vi "duplicate channel.vi"(8 "number of available channels":u16, 11 "Sensor List":u32) -> (2 "Sensor Array out":T1, 3 "IndexVals":u32)   [LabVIEW 2015]
uses:
  DAQ configuration/Sensor array.ctl
  DAQ configuration/channel identifier.ctl
  DAQ configuration/Sensor buffer command.ctl
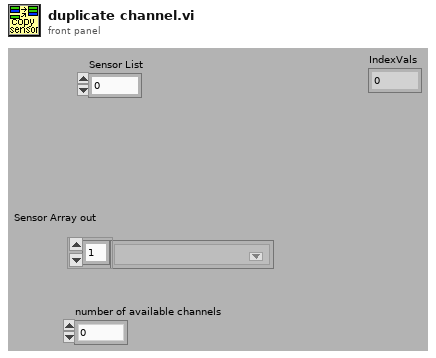
[diagram p1: front panel]
types:
  T1 = typedef "Sensor array.ctl" = T2[]
  T2 = typedef "channel identifier.ctl" = u16
  T3 = typedef "Sensor buffer command.ctl" = enum16{"read average", "read recent", "read all", "write", "set buffer size", "Read channel config", "Write channel config", "clear"}
  T4 = typedef "Channel config.ctl" = cluster{"Channel Indices":T2[], "AI Max voltage":dbl[], "Calibration matrix":T5}
  T5 = typedef "calib array.ctl" = T6[]
  T6 = typedef "conversion.ctl" = cluster{"conversion matrix":sgl[][], "units":string, "name":string, "scale type":T7, "offset (volts)":dbl, "second channel":i8, "correspondence table":T8, "offset (physical units)":dbl, "pH scale":T9, "D.O.":T10, "Photometer data":T11}
  T7 = typedef "scale type.ctl" = enum16{"Volts", "Polynomial", "Correspondence Table", "pH", "Dissolved Oxygen", "Quadratic", "Photometer"}
  T8 = typedef "correspondence table.ctl" = cluster{"physical units":dbl, "volts":dbl}[]
  T9 = typedef "pH scale.ctl" = cluster{"Buffers":cluster{"Buffer":dbl, "Calibrated":bool, "V/T":dbl}[], "Temperature":dbl}
  T10 = typedef "DO scale.ctl" = cluster{"Temperature":dbl, "K":dbl, "barometric pressure":dbl}
  T11 = typedef "Photometer calibration data.ctl" = cluster{"Dark Voltage":dbl, "Blank Voltage":dbl, "Standards":cluster{"Concentration":dbl, "Voltage":dbl}[]}
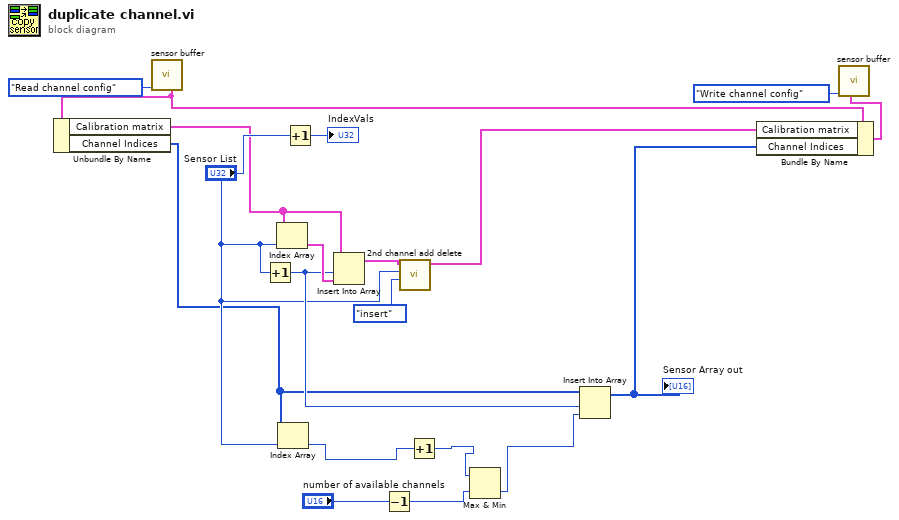
[diagram p0: block diagram]
diagram:
  n1 = call "sensor buffer.vi"("command"=Sensor_buffer_command."Read channel config") -> ("Channel Config out"=w7:T4)  [unwired: 6 in, 4 out]
  n2 = Unbundle By Name(w7) -> ("Calibration matrix"=w6:T5, "Channel Indices"=w3:T2[])
  n3 = Increment(x="Sensor List") -> (x+1=w18:u32)
  n4 = Index Array(array=w6, index="Sensor List") -> (element=w19:T6)
  n5 = Index Array(array=w3, index="Sensor List") -> (element=w13:T2)
  n6 = Increment(x="Sensor List") -> (x+1=→"IndexVals":u32)
  n7 = Insert Into Array(array=w6, index=w18, new element=w19) -> (w17:T5)
  n8 = Decrement(x="number of available channels") -> (x-1=w1:u16)
  n9 = call "2nd channel add delete.vi"("action"=enum16{"delete", "insert"}."insert", "Index"="Sensor List", "Calibration array"=w17) -> ("Calibration array out"=w5:T5)  [unwired: 8 in]
  n10 = Increment(x=w13) -> (x+1=w11:T2)
  n11 = Max & Min(x=w11, y=w1) -> (min(x,y)=w10:T2)  [unwired: 1 out]
  n12 = Insert Into Array(array=w3, index=w18, new element=w10) -> (w4:T2[])
  "Sensor Array out" <- w4
  n13 = Bundle By Name(cluster=w7, "Calibration matrix"=w5, "Channel Indices"=w4) -> (w2:T4)
  n14 = call "sensor buffer.vi"("Channel Config"=w2, "command"=Sensor_buffer_command."Write channel config") -> ()  [unwired: 5 in, 5 out]
